vi "Interface1.1.vi"() -> ()   [LabVIEW 2016]
uses:
  <vilib>/userdefined/High Color/IMAQdx.ctl
  System.Speech
  <vilib>/vision/driver/NI_Vision_Acquisition_Software.lvlib
  <vilib>/vision/NI_Vision_Development_Module.lvlib
  <resource>/objmgr/imaqdx.rc
panel:
  in  "Tab Control":enum32{"Page 1", "Page 2"}(tab)
  out "Read String":string
  out "Image 5":T1(plugin-control)
  in  "File Path":path
  in  "Rectangle":T2 {"Rotation" min=-90.0 max=90.0 step=1.0 format="%.2f"; "Left" scale=0.0..1024.0; "Right" scale=0.0..1024.0}
  out "Cam":T1(plugin-control)
  out "5":string
  out "4":string
  out "3":string
  out "2":string
  out "1":string
  in  "stop":bool
  out "Cam0":T1(plugin-control)
  out "concatenated string":string
  out "l":bool
  out "a":bool
  out "s":bool
  out "u":bool
  out "Image":T1(plugin-control)
  out "Image 2":T1(plugin-control)
  out "Image 3":T1(plugin-control)
  out "Image 4":T1(plugin-control)
  out "Image 7":T1(plugin-control)
  out "t":bool
  out "Number of Matches":i32
  in  "Image Type":T3 items=["Grayscale (U8)", "Grayscale (I16)", "Grayscale (SGL)", "Complex (CSG)", "RGB (U32)", "HSL (U32)", "RGB (U64)", "Grayscale (U16)"]
  out "error IO":errorcluster
  # "Choose an option click on \n         Page 1 if you want hand recognition\n         Page 2 if u want OCR"
  # "zd"
  # "sk"
  # "dd"
  # "lllss"
  # "Output String"
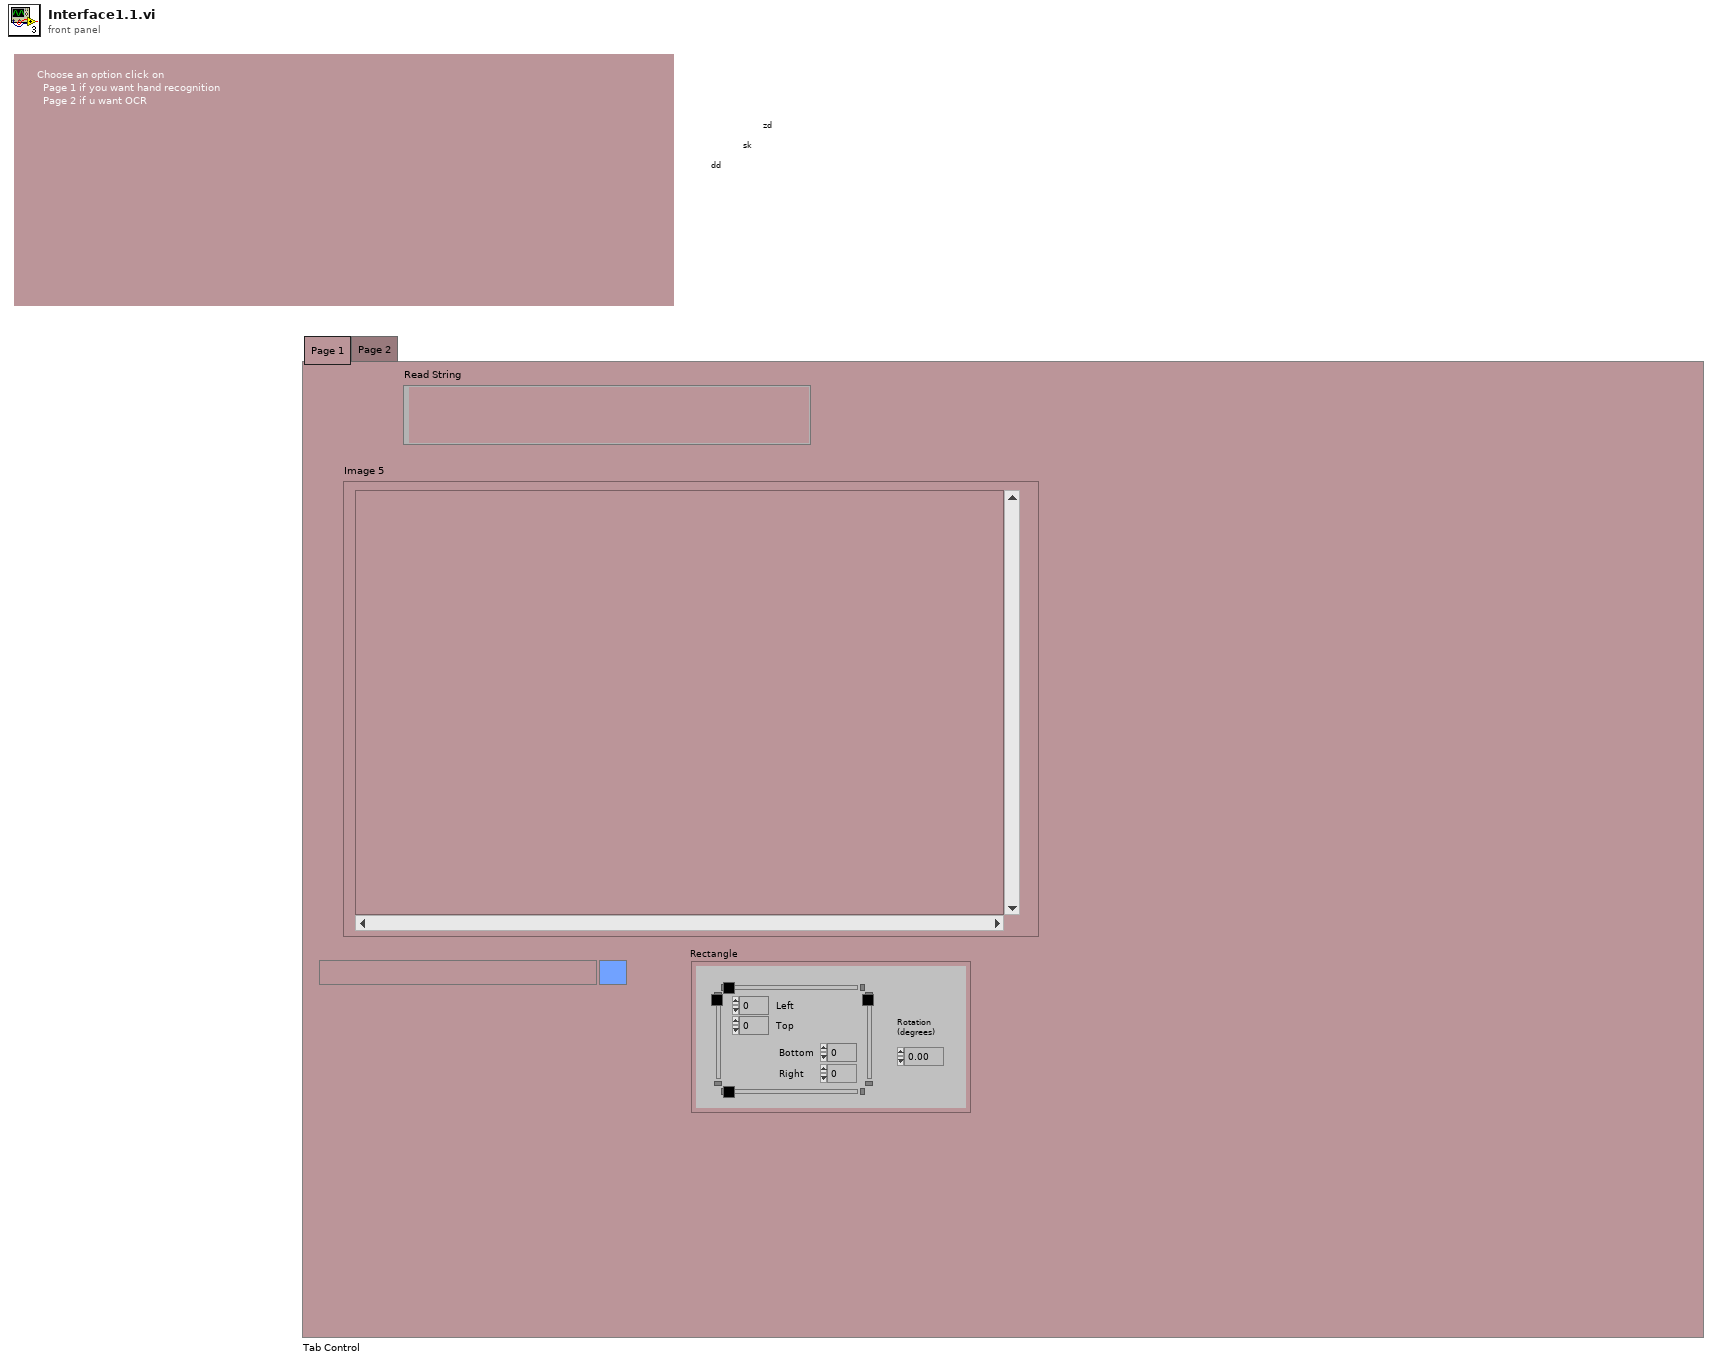
[diagram p1: front panel]
types:
  T1 = typedef "IMAQ Image.ctl" = refnum<image>
  T2 = typedef "IMAQ Rectangle" = cluster{"Left":i32, "Top":i32, "Right":i32, "Bottom":i32, "Rotation":dbl}
  T3 = typedef "Image Type" = u32
  T4 = typedef "IMAQdx.ctl" = refnum<k21>
  T5 = enum32{"AutoM", "Close", "Dilate", "Erode", "Gradient", "Gradient in", "Gradient out", "HitMiss", "Open", "PClose", "POpen", "Thick", "Thin"}
  T6 = typedef "IMAQ OCR Session.ctl" = refnum<k1>
  T7 = typedef "ROI Descriptor" = cluster{"Global Rectangle":i32[], "Contours":cluster{"ID":enum32{"External", "Internal"}, "Type":u32, "Coordinates":i32[]}[]}
  T8 = cluster{"Global Rectangle":i32[], "Contours":cluster{"ID":enum32{"External", "Internal"}, "Type":u32, "Coordinates":i32[]}[]}
  T9 = cluster{"Position":cluster{"x":sgl, "y":sgl}, "Angle":sgl, "Scale":sgl, "Score":sgl, "Bounding Box":cluster{"x":sgl, "y":sgl}[]}[]
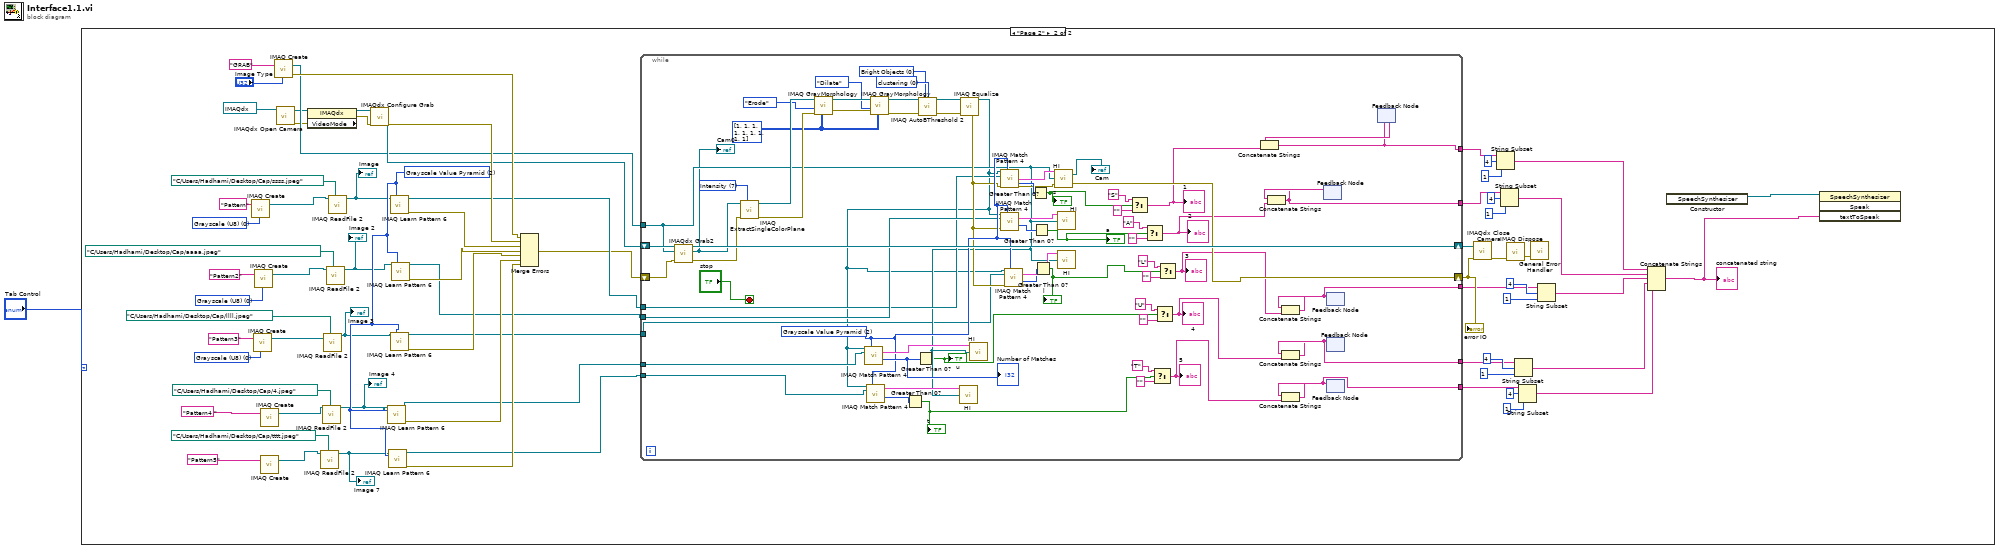
[diagram p0: block diagram]
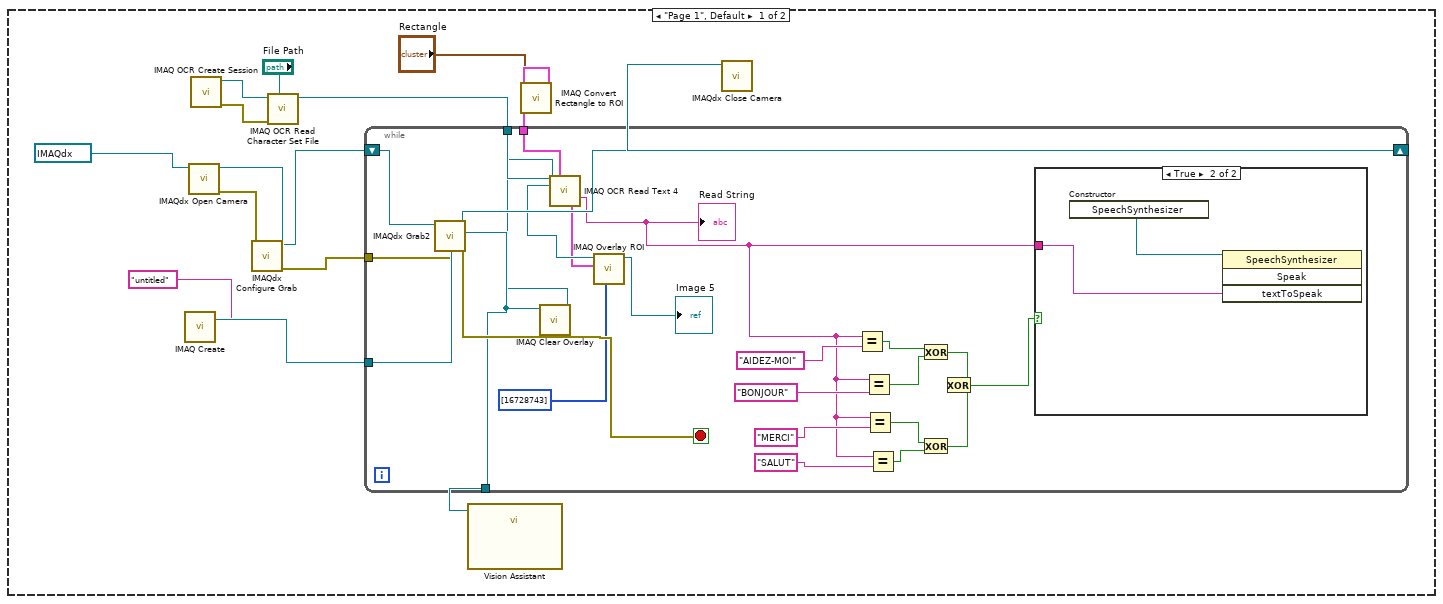
[diagram p2: hidden frame]
diagram:
  n1 = case shown="\"Page 2\"" "Tab Control" {
    frame "Page 1", Default {
      n2 = call "IMAQ Create"("Image Name"="untitled") -> ("New Image"=w13:T1)  [unwired: 4 in, 1 out]
      n3 = call <vilib>:"IMAQdx Open Camera.vi"("Session In"=T4 "cam0") -> ("error out"=w15:errorcluster, "Session Out"=w16:T4)  [unwired: 9 in]
      n4 = call "IMAQ OCR Create Session"() -> ("error out"=w6:errorcluster, "IMAQ OCR Session"=w7:T6)  [unwired: 10 in]
      n5 = call <vilib>:"IMAQdx Configure Grab.vi"("error in"=w15, "Session In"=w16) -> ("error out"=w9:errorcluster, "Session Out"=w14:T4)  [unwired: 8 in]
      n6 = call "IMAQ OCR Read Character Set File"("File Path"="File Path", "error in (no error)"=w6, "IMAQ OCR Session"=w7) -> ("IMAQ OCR Session (dup)"=w5:T6)  [unwired: 6 in, 2 out]
      n7 = call "IMAQ Convert Rectangle to ROI"("Rectangle"="Rectangle") -> ("ROI Descriptor"=w4:T7)  [unwired: 8 in, 1 out]
      n8 = while {
        tunnel: w13 -> [w40]
        shift-right: [w39] -> w11
        shift-left: w14 -> [w41]
        tunnel: w9 -> [w38]
        tunnel: w5 -> [w37]
        tunnel: w4 -> [w36]
        tunnel: [w32] -> w2
        stop <- w35 stop-if-true
        n9 = call <vilib>:"IMAQdx Grab2.vi"("error in"=w38, "Image In"=w40, "Session In"=w41) -> ("error out"=w35:errorcluster, "Image Out"=w32:T1, "Session Out"=w39:T4)  [unwired: 5 in, 1 out]
        n10 = call "IMAQ Clear Overlay"("Image"=w32) -> ("Image Out"=w31:T1)  [unwired: 9 in, 1 out]
        n11 = call "IMAQ OCR Read Text 4"("IMAQ OCR Session"=w37, "ROI Descriptor"=w36, "Image"=w31) -> ("Image (dup)"=w34:T1, "Read String"=w18:string, "ROI Bounding Characters"=w33:T8)  [unwired: 6 in, 4 out]
        "Read String" <- w18
        n12 = call "IMAQ Overlay ROI"("Colors (Green)"=u32[] [16728743], "ROI Descriptor"=w33, "Image"=w34) -> ("Image Out"=→"Image 5":T1)  [unwired: 7 in, 1 out]
        n13 = Equal?(x=w18, y="AIDEZ-MOI") -> (x = y?=w24:bool)
        n14 = Equal?(x=w18, y="BONJOUR") -> (x = y?=w23:bool)
        n15 = Equal?(x=w18, y="MERCI") -> (x = y?=w22:bool)
        n16 = Equal?(x=w18, y="SALUT") -> (x = y?=w21:bool)
        n17 = Exclusive Or(1:w23, 2:w24) -> (0:w19:bool)
        n18 = Exclusive Or(1:w21, 2:w22) -> (0:w20:bool)
        n19 = Exclusive Or(1:w20, 2:w19) -> (0:w17:bool)
        n20 = case shown="True" w17 {
          tunnel: w18 -> [_ w42]
          frame False {
          }
          frame True {
            n21 = constructor class="SpeechSynthesizer"() -> (reference out=w43:refnum<k24>)  [unwired: 3 in, 2 out]
            n22 = invoke class="SpeechSynthesizer" method="Speak"(reference=w43, "textToSpeak"=w42) -> ()  [unwired: 2 in, 4 out]
          }
        }
      }
      n23 = call "Vision Assistant"("Image In"=w2) -> ()  [unwired: 25 in, 2 out]
      n24 = call <vilib>:"IMAQdx Close Camera.vi"("Session In"=w11) -> ()  [unwired: 10 in, 1 out]
    }
    frame "Page 2" {
      w97 = 2 items=["All", "Low Discrepancy Sampling", "Grayscale Value Pyramid", "Gradients Pyramid"] ("Algorithm")
      w107 = T3 0 items=["Grayscale (U8)", "Grayscale (I16)", "Grayscale (SGL)", "Complex (CSG)", "RGB (U32)", "HSL (U32)", "RGB (U64)", "Grayscale (U16)"] ("Image Type")
      w108 = T3 0 items=["Grayscale (U8)", "Grayscale (I16)", "Grayscale (SGL)", "Complex (CSG)", "RGB (U32)", "HSL (U32)", "RGB (U64)", "Grayscale (U16)"] ("Image Type")
      w109 = T3 0 items=["Grayscale (U8)", "Grayscale (I16)", "Grayscale (SGL)", "Complex (CSG)", "RGB (U32)", "HSL (U32)", "RGB (U64)", "Grayscale (U16)"] ("Image Type")
      n25 = call "IMAQ Create"("Image Name"="Pattern", "Image Type"=w109) -> ("New Image"=w106:T1)  [unwired: 3 in, 1 out]
      n26 = call "IMAQ Create"("Image Name"="Pattern3", "Image Type"=w107) -> ("New Image"=w104:T1)  [unwired: 3 in, 1 out]
      n27 = call "IMAQ Create"("Image Name"="Pattern2", "Image Type"=w108) -> ("New Image"=w105:T1)  [unwired: 3 in, 1 out]
      n28 = call "IMAQ Create"("Image Name"="Pattern4 ") -> ("New Image"=w66:T1)  [unwired: 4 in, 1 out]
      n29 = call "IMAQ Create"("Image Name"="Pattern5") -> ("New Image"=w98:T1)  [unwired: 4 in, 1 out]
      n30 = call "IMAQ Create"("Image Name"="GRAB", "Image Type"="Image Type") -> ("New Image"=w80:T1, "error out"=w93:errorcluster)  [unwired: 3 in]
      n31 = call <vilib>:"IMAQdx Open Camera.vi"("Session In"=T4 "cam0") -> ("error out"=w76:errorcluster, "Session Out"=w74:T4)  [unwired: 9 in]
      n32 = property class="IMAQdx" props=["VideoMode"](reference=w74, error in=w76) -> (reference out=w73:T4, error out=w75:errorcluster)  [unwired: 1 out]
      n33 = call "IMAQ ReadFile 2"("File Path"=path "C:/Users/Hadhami/Desktop/Cap/tttt.jpeg", "Image"=w98) -> ("Image Out"=w67:T1)  [unwired: 5 in, 4 out]
      "Image 7" <- w67
      n34 = call "IMAQ ReadFile 2"("File Path"=path "C:/Users/Hadhami/Desktop/Cap/4.jpeg", "Image"=w66) -> ("Image Out"=w68:T1)  [unwired: 5 in, 4 out]
      "Image 4" <- w68
      n35 = call "IMAQ ReadFile 2"("File Path"=path "C:/Users/Hadhami/Desktop/Cap/llll.jpeg", "Image"=w104) -> ("Image Out"=w69:T1)  [unwired: 5 in, 4 out]
      "Image 3" <- w69
      n36 = call "IMAQ ReadFile 2"("File Path"=path "C:/Users/Hadhami/Desktop/Cap/aaaa.jpeg", "Image"=w105) -> ("Image Out"=w70:T1)  [unwired: 5 in, 4 out]
      "Image 2" <- w70
      n37 = call "IMAQ ReadFile 2"("File Path"=path "C:/Users/Hadhami/Desktop/Cap/ssss.jpeg", "Image"=w106) -> ("Image Out"=w71:T1)  [unwired: 5 in, 4 out]
      "Image" <- w71
      n38 = call <vilib>:"IMAQdx Configure Grab.vi"("error in"=w75, "Session In"=w73) -> ("error out"=w94:errorcluster, "Session Out"=w81:T4)  [unwired: 8 in]
      n39 = call "IMAQ Learn Pattern 6"("Image"=w68, "Algorithm"=w97) -> ("Template Image Out"=w86:T1, "error out"=w96:errorcluster)  [unwired: 11 in, 1 out]
      n40 = call "IMAQ Learn Pattern 6"("Image"=w67, "Algorithm"=w97) -> ("Template Image Out"=w87:T1, "error out"=w95:errorcluster)  [unwired: 11 in, 1 out]
      n41 = call "IMAQ Learn Pattern 6"("Image"=w71, "Algorithm"=w97) -> ("Template Image Out"=w83:T1, "error out"=w103:errorcluster)  [unwired: 11 in, 1 out]
      n42 = call "IMAQ Learn Pattern 6"("Image"=w69, "Algorithm"=w97) -> ("Template Image Out"=w85:T1, "error out"=w101:errorcluster)  [unwired: 11 in, 1 out]
      n43 = call "IMAQ Learn Pattern 6"("Image"=w70, "Algorithm"=w97) -> ("Template Image Out"=w84:T1, "error out"=w102:errorcluster)  [unwired: 11 in, 1 out]
      n44 = Merge Errors(w93, w94, w103, w102, w101, w96, w95) -> (w82:errorcluster)
      n45 = while {
        tunnel: w87 -> [w173]
        tunnel: w86 -> [w172]
        tunnel: w85 -> [w150]
        tunnel: w84 -> [w154]
        tunnel: w83 -> [w153]
        shift-right: [w185] -> w79
        shift-left: w81 -> [w187]
        tunnel: w80 -> [w152]
        shift-right: [w155] -> w72
        shift-left: w82 -> [w186]
        tunnel: [w116] -> w65
        tunnel: [w120] -> w54
        tunnel: [w119] -> w53
        tunnel: [w118] -> w52
        tunnel: [w117] -> w51
        stop <- "stop" stop-if-true
        w158 = u32 0 items=["Bright Objects", "Dark Objects"] ("Look For (Bright Objects)")
        w159 = 0 items=["clustering", "entropy", "metric", "moments", "inter-class variance"] ("Method (clustering)")
        w160 = 7 items=["Red", "Green", "Blue", "Hue", "Saturation", "Luminance", "Value", "Intensity"] ("Color Plane")
        w161 = 2 items=["All", "Low Discrepancy Sampling", "Grayscale Value Pyramid", "Gradients Pyramid"] ("Algorithm")
        w174 = i32[][] [[1, 1, 1], [1, 1, 1], [1, 1, 1]] ("Structuring Element")
        n46 = call <vilib>:"IMAQdx Grab2.vi"("error in"=w186, "Image In"=w152, "Session In"=w187) -> ("error out"=w149:errorcluster, "Image Out"=w151:T1, "Session Out"=w185:T4)  [unwired: 5 in, 1 out]
        "Cam0" <- w151
        n47 = call "IMAQ ExtractSingleColorPlane"("Color Plane"=w160, "error in (no error)"=w149, "Image Src"=w151) -> ("error out"=w184:errorcluster, "Image Dst Out"=w183:T1)  [unwired: 7 in]
        n48 = call "IMAQ GrayMorphology"("Structuring Element"=w174, "error in (no error)"=w184, "Operation"=T5."Erode", "Image Src"=w183) -> ("error out"=w182:errorcluster, "Image Dst Out"=w181:T1)  [unwired: 6 in]
        n49 = call "IMAQ GrayMorphology"("Structuring Element"=w174, "error in (no error)"=w182, "Operation"=T5."Dilate", "Image Src"=w181) -> ("error out"=w178:errorcluster, "Image Dst Out"=w180:T1)  [unwired: 6 in]
        n50 = call "IMAQ AutoBThreshold 2"("Image Src"=w180, "Look For (Bright Objects)"=w158, "Method (clustering)"=w159, "error in (no error)"=w178) -> ("Image Dst Out"=w179:T1, "error out"=w177:errorcluster)  [unwired: 9 in, 1 out]
        n51 = call "IMAQ Equalize"("error in (no error)"=w177, "Image Src"=w179) -> ("error out"=w157:errorcluster, "Image Dst Out"=w147:T1)  [unwired: 8 in]
        n52 = call "IMAQ Match Pattern 4"("Image"=w147, "Algorithm"=w161, "Template Image"=w172) -> ("Matches (pixel)"=w169:T9, "Number of Matches"=w168:i32)  [unwired: 8 in, 3 out]
        "Number of Matches" <- w168
        n53 = call "IMAQ Match Pattern 4"("Image"=w147, "Algorithm"=w161, "Template Image"=w173) -> ("Matches (real-world)"=w171:T9, "Number of Matches"=w170:i32)  [unwired: 8 in, 3 out]
        n54 = Greater Than 0?(x=w170) -> (x > 0?=w137:bool)
        "t" <- w137
        n55 = Greater Than 0?(x=w168) -> (x > 0?=w139:bool)
        "u" <- w139
        n56 = call "HI.vi"("Image"=w152, "Matches (pixel)"=w171) -> ()  [unwired: 1 in, 2 out]
        n57 = call "HI.vi"("Image"=w152, "Matches (pixel)"=w169) -> ()  [unwired: 1 in, 2 out]
        n58 = call "IMAQ Match Pattern 4"("Image"=w147, "Algorithm"=w161, "Template Image"=w153, "error in (no error)"=w157) -> ("Matches (pixel)"=w162:T9, "Number of Matches"=w165:i32, "error out"=w156:errorcluster)  [unwired: 7 in, 2 out]
        n59 = call "IMAQ Match Pattern 4"("Image"=w147, "Algorithm"=w161, "Template Image"=w154, "error in (no error)"=w157) -> ("Matches (pixel)"=w166:T9, "Number of Matches"=w164:i32)  [unwired: 7 in, 3 out]
        n60 = call "IMAQ Match Pattern 4"("Image"=w147, "Algorithm"=w161, "Template Image"=w150, "error in (no error)"=w157) -> ("Matches (pixel)"=w167:T9, "Number of Matches"=w163:i32)  [unwired: 7 in, 3 out]
        n61 = Greater Than 0?(x=w165) -> (x > 0?=w146:bool)
        "s" <- w146
        n62 = Greater Than 0?(x=w164) -> (x > 0?=w143:bool)
        "a" <- w143
        n63 = Greater Than 0?(x=w163) -> (x > 0?=w141:bool)
        "l" <- w141
        n64 = call "HI.vi"("error in (no error)"=w156, "Image"=w152, "Matches (pixel)"=w162) -> ("error out"=w155:errorcluster, "Image Out"=→"Cam":T1)
        n65 = call "HI.vi"("Image"=w152, "Matches (pixel)"=w166) -> ()  [unwired: 1 in, 2 out]
        n66 = call "HI.vi"("Image"=w152, "Matches (pixel)"=w167) -> ()  [unwired: 1 in, 2 out]
        n67 = Select(t="S", s=w146, f="") -> (s? t:f=w125:string)
        "1" <- w125
        n68 = Select(t="A", s=w143, f="") -> (s? t:f=w124:string)
        "2" <- w124
        n69 = Select(t="T", s=w137, f="") -> (s? t:f=w121:string)
        "5" <- w121
        n70 = Select(t="U", s=w139, f="") -> (s? t:f=w122:string)
        "4" <- w122
        n71 = Select(t="L", s=w141, f="") -> (s? t:f=w123:string)
        "3" <- w123
        n72 = feedback #1() -> (w129:string)  [unwired: 1 in]
        n73 = Concatenate Strings(w129, w124) -> (w117:string)
        n74 = feedback-in #1(w117) -> ()
        n75 = feedback #2() -> (w118:string)  [unwired: 1 in]
        n76 = Concatenate Strings(w118, w123) -> (w130:string)
        n77 = feedback-in #2(w130) -> ()
        n78 = feedback #3() -> (w127:string)  [unwired: 1 in]
        n79 = Concatenate Strings(w127, w122) -> (w119:string)
        n80 = feedback-in #3(w119) -> ()
        n81 = feedback #4() -> (w120:string)  [unwired: 1 in]
        n82 = Concatenate Strings(w120, w121) -> (w126:string)
        n83 = feedback-in #4(w126) -> ()
        n84 = feedback #5() -> (w128:string)  [unwired: 1 in]
        n85 = Concatenate Strings(w128, w125) -> (w116:string)
        n86 = feedback-in #5(w116) -> ()
      }
      "error IO" <- w72
      n87 = call <vilib>:"IMAQdx Close Camera.vi"("error in"=w72, "Session In"=w79) -> ("error out"=w78:errorcluster)  [unwired: 9 in]
      n88 = String Subset(string=w65, offset (0)=4, length (rest)=1 ("length (rest)")) -> (substring=w50:string)
      n89 = String Subset(string=w51, offset (0)=4, length (rest)=1 ("length (rest)")) -> (substring=w49:string)
      n90 = call "IMAQ Dispose"("error in (no error)"=w78) -> ("error out"=w77:errorcluster)  [unwired: 5 in]
      n91 = String Subset(string=w53, offset (0)=4, length (rest)=1 ("length (rest)")) -> (substring=w47:string)
      n92 = String Subset(string=w54, offset (0)=4, length (rest)=1 ("length (rest)")) -> (substring=w46:string)
      n93 = call <vilib>:"General Error Handler.vi"("error in (no error)"=w77) -> ()  [unwired: 10 in, 5 out]
      n94 = String Subset(string=w52, offset (0)=4, length (rest)=1 ("length (rest)")) -> (substring=w48:string)
      n95 = Concatenate Strings(w50, w49, w48, w47, w46) -> (w44:string)
      "concatenated string" <- w44
      n96 = constructor class="SpeechSynthesizer"() -> (reference out=w45:refnum<k24>)  [unwired: 3 in, 2 out]
      n97 = invoke class="SpeechSynthesizer" method="Speak"(reference=w45, "textToSpeak"=w44) -> ()  [unwired: 2 in, 4 out]
    }
  }
